vi "Logout.vi"(7 "Values In":refnum<class "Values.lvclass">, 8 "error in (no error)":errorcluster, 10 "Session In":refnum<class "Session.lvclass">, 11 "Security in":refnum<class "Security.lvclass">) -> (0 "error out":errorcluster, 2 "Session":refnum<class "Session.lvclass">, 3 "Security out":refnum<class "Security.lvclass">, 5 "Values":refnum<class "Values.lvclass">)   [LabVIEW 2020, in "HTTP Server.lvlib" / "Security.lvclass"]
uses:
  Security.lvclass
  Session/Session.lvclass
  Values/Values.lvclass
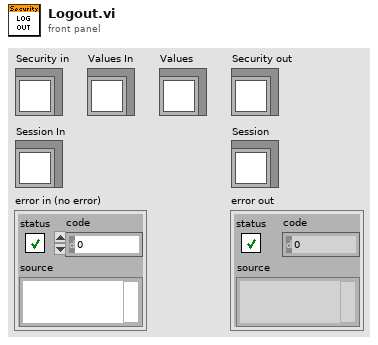
[diagram p1: front panel]
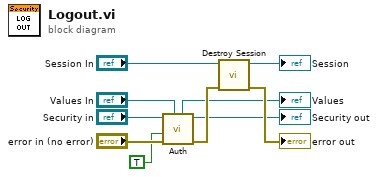
[diagram p0: block diagram]
diagram:
  n1 = call "Auth.vi"("Values In"="Values In", "error in (no error)"="error in (no error)", "Anonymous (F)"=TRUE, "Security in"="Security in") -> ("error out"=w9:errorcluster, "Security out"=→"Security out":refnum<class "Security.lvclass">, "Values"=→"Values":refnum<class "Values.lvclass">)  [unwired: 5 in]
  n2 = call "Destroy Session.vi"("error in (no error)"=w9, "Session in"="Session In") -> ("error out"=→"error out":errorcluster, "Session out"=→"Session":refnum<class "Session.lvclass">)  [unwired: 8 in]
